vi "Open TCP Connection.vi"(8 "error in (no error)":errorcluster, 11 "MJPEG Reader in":refnum<class "MJPEG Reader.lvclass">) -> (0 "error out":errorcluster, 3 "MJPEG Reader out":refnum<class "MJPEG Reader.lvclass">)   [LabVIEW 2015, in "MJPEG Reader.lvclass"]
uses:
  MJPEG Reader.lvclass
  MJPEG Reader.lvclass/MJPEG Reader.ctl
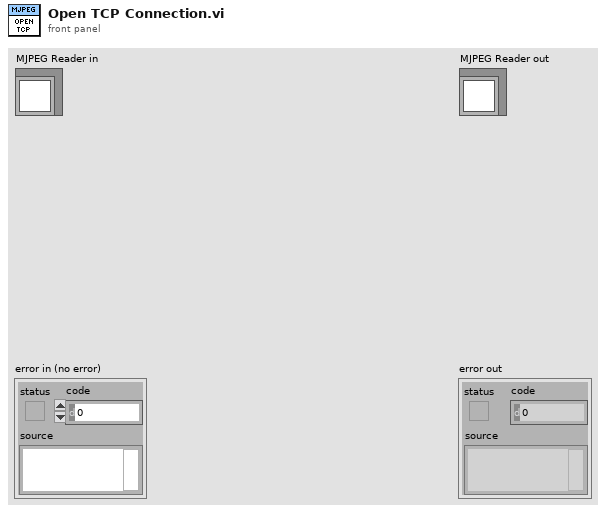
[diagram p1: front panel]
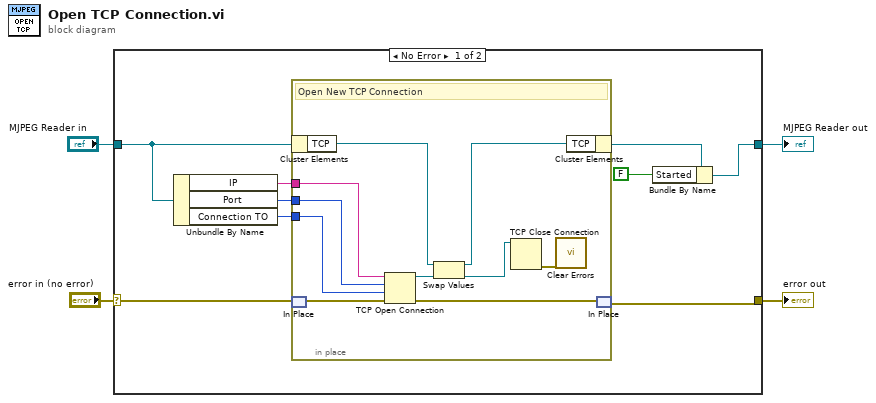
[diagram p0: block diagram]
diagram:
  n1 = case shown="No Error" "error in (no error)" {
    selector: "error in (no error)" -> [w13 w25]
    tunnel: [w8 w25] -> w3
    tunnel: [w6 w24] -> w1
    tunnel: "MJPEG Reader in" -> [w12 w24]
    frame No Error {
      n2 = Unbundle By Name(w12) -> ("IP"=w11:string, "Port"=w10:u16, "Connection TO"=w9:i32)
      n3 = in-place {
        in-place-border: w11 -> [w21]
        in-place-border: w10 -> [w20]
        in-place-border: w9 -> [w19]
        # "Open New TCP Connection"
        n4 = in-place-cluster #1(w12) -> ("TCP"=w16:refnum<k5>)
        n5 = in-place-match #2(w13) -> (w22:errorcluster)
        n6 = TCP Open Connection(address=w21, remote port or service name=w20, timeout ms (60000)=w19, error in (no error)=w22) -> (connection ID=w18:refnum<k5>, error out=w17:errorcluster)  [unwired: 1 in]
        n7 = Swap Values(12:w16, 14:w18) -> (1:w23:refnum<k5>, 3:w15:refnum<k5>)  [unwired: 1 in]
        n8 = TCP Close Connection(connection ID=w15) -> (error out=w14:errorcluster)  [unwired: 2 in, 1 out]
        n9 = call <vilib>:"Clear Errors.vi"("error in (no error)"=w14) -> ()  [unwired: 5 in, 2 out]
        n10 = in-place-cluster #1("TCP"=w23) -> (w7:refnum<class "MJPEG Reader.lvclass">)
        n11 = in-place-match #2(w17) -> (w8:errorcluster)
      }
      n12 = Bundle By Name(cluster=w7, "Started"=FALSE) -> (w6:refnum<class "MJPEG Reader.lvclass">)
    }
    frame Error {
    }
  }
  "error out" <- w3
  "MJPEG Reader out" <- w1
